vi "同步RS触发器（与非门）.vi"(1 "R":bool, 2 "CP":bool, 3 "S":bool) -> (0 "Q":bool)   [LabVIEW 2012, in "触发器.lvlib"]
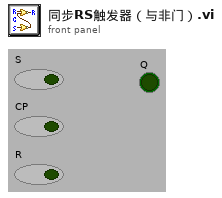
[diagram p1: front panel]
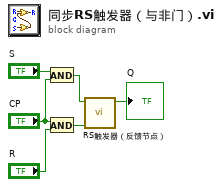
[diagram p0: block diagram]
diagram:
  n1 = And(x="S", y="CP") -> (x .and. y?=w3:bool)
  n2 = And(x="CP", y="R") -> (x .and. y?=w2:bool)
  n3 = call "RS触发器（反馈节点）.vi"("R"=w2, "S"=w3) -> ("Q"=→"Q":bool)  [unwired: 9 in]
